vi "Resize Panel to Pane.vi"(8 "error in (no error)":errorcluster, 10 "NewBnds":T1, 11 "IViewManager In":refnum<class "IViewManager.lvclass">) -> (0 "error out":errorcluster, 3 "IViewManager Out":refnum<class "IViewManager.lvclass">)   [LabVIEW 2015, in "IViewManager.lvlib" / "IViewManager.lvclass"]
uses:
  IViewManager.lvclass
  <vilib>/Utility/miscctls.llb/LVRectTypeDef.ctl
  IViewManager.lvclass/IViewManager.ctl
  IViewable/IViewable Messages/Resize Panel to Pane Msg/Resize Panel to Pane Msg.lvclass/Resize Panel to Pane Msg.ctl
  <vilib>/ActorFramework/Message Enqueuer/Message Enqueuer.lvclass/Message Enqueuer.ctl
  <vilib>/ActorFramework/Message Enqueuer/Enqueue.vi
  <vilib>/ActorFramework/Message Priority Queue/Priority Enqueue.vi
  IViewable/IViewable/IViewable.lvclass
  IViewable/IViewable Messages/Resize Panel to Pane Msg/Resize Panel to Pane Msg.lvclass
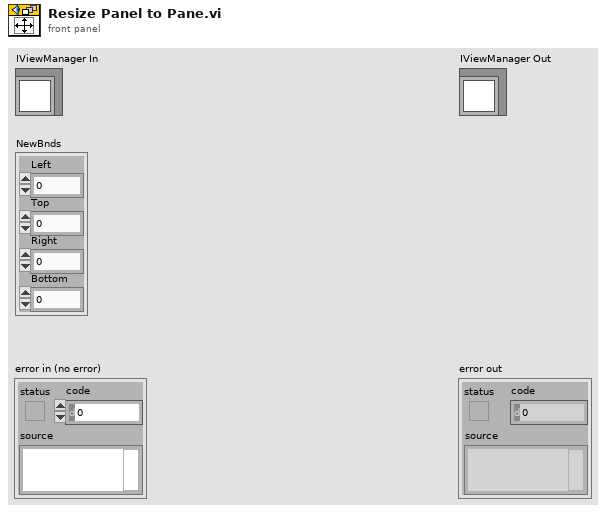
[diagram p1: front panel]
types:
  T1 = typedef "LVRectTypeDef.ctl" = cluster{"Left":i16, "Top":i16, "Right":i16, "Bottom":i16}
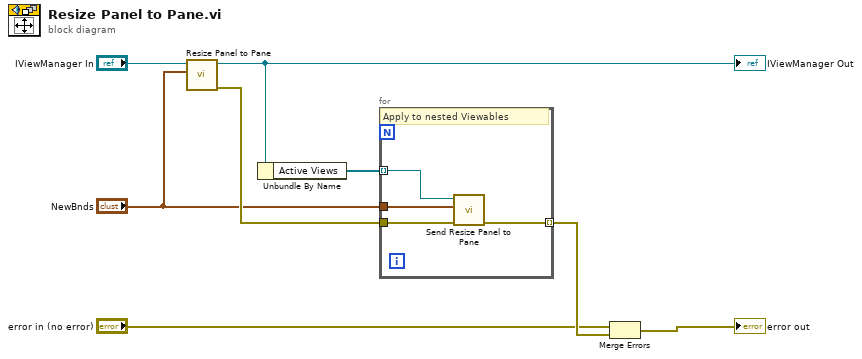
[diagram p0: block diagram]
diagram:
  n1 = call-parent "Resize Panel to Pane.vi"("NewBnds"="NewBnds", "IViewable In"="IViewManager In") -> ("error out"=w8:errorcluster, "IViewable Out"=w2:refnum<class "IViewManager.lvclass">)  [unwired: 8 in]
  "IViewManager Out" <- w2
  n2 = Unbundle By Name(w2) -> ("Active Views"=w6:refnum<class "Message Enqueuer.lvclass">[])
  n3 = for {
    tunnel: w6 -> [w12] mode=indexing
    tunnel: w8 -> [w11]
    tunnel: [w10] -> w7 mode=indexing
    tunnel: "NewBnds" -> [w9]
    # "Apply to nested Viewables"
    n4 = call "Send Resize Panel to Pane.vi"("error in (no error)"=w11, "NewBnds"=w9, "Message Enqueuer"=w12) -> ("error out"=w10:errorcluster)  [unwired: 7 in, 1 out]
  }
  n5 = Merge Errors("error in (no error)", w7) -> (→"error out":errorcluster)
